vi "PIM Configuration.vi"(6 "Write? (f)":bool, 7 "Connection Refnum":T2, 8 "error in (no error)":errorcluster, 9 "Configuration (\"\")":string, 11 "Template Keys (empty)":T1) -> (0 "error out":errorcluster, 1 "Configuration":string, 3 "Template Keys":T1, 5 "Connection Refnum":T2)   [LabVIEW 2011]
uses:
  ITK/utils/keyedarr.llb/Keyed Array.ctl
  ITK/utils/strutil.llb/Case Matching.ctl
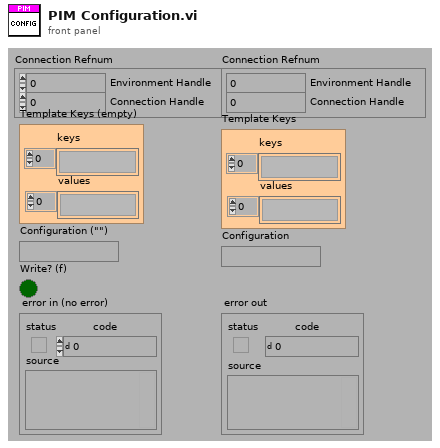
[diagram p1: front panel]
types:
  T1 = typedef "Keyed Array.ctl" = cluster{"keys":string[], "values":string[]}
  T2 = cluster{"Environment Handle":i32, "Connection Handle":i32}
  T3 = typedef "Case Matching.ctl" = enum16{"a != A", "a == A", "system"}
  T4 = typedef "PIM Test Parameters.ctl" = cluster{"Stimulus":T5, "Measure":T7, "Display":T13}
  T5 = typedef "PIM Stimulus Parameters.ctl" = cluster{"C1 Pwr dBm":dbl, "C2 Pwr dBm":dbl, "Power Units":enum16{"dBm", "Watts"}, "Meas Type":enum32{"Time", "Frequency"}, "C1 Freq MHz":dbl, "C2 Freq MHz":dbl, "Swept Freq Step":T6}
  T6 = typedef "PIM Sweep Step Size.ctl" = u16
  T7 = typedef "PIM Measurement Parameters.ctl" = cluster{"IM Order":T8, "Direction":T9, "Averaging":T10, "ALC ON?":bool, "Peak Hold?":bool, "Peak last N":u32, "Ref Level dBm":dbl, "Ref Units":enum16{"dBm", "dBc"}, "Num Samples":u32, "Sample units":T11, "Update Rate (s)":dbl, "DUT PORT":T12, "Percent (%)":u8}
  T8 = typedef "IMOrder.ctl" = u8
  T9 = typedef "MeasMode.ctl" = u16
  T10 = typedef "HW Averaging.ctl" = u16
  T11 = typedef "PIM Meas Units.ctl" = enum16{"Sample(s)", "Second(s)", "Sweep(s)"}
  T12 = typedef "DUTport.ctl" = enum16{"Port 1", "Port 2"}
  T13 = typedef "PIM Display Parameters.ctl" = cluster{"Power Scale":cluster{"yRange_min":i32, "yRange_max":i32}, "xRange_span":u32}
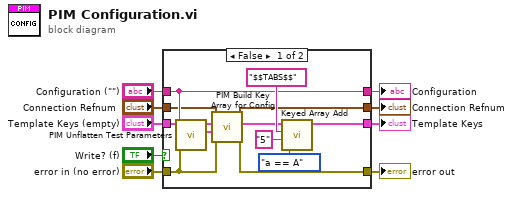
[diagram p0: block diagram]
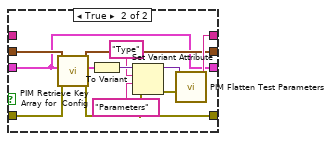
[diagram p2: hidden frame]
diagram:
  n1 = case shown="False" "Write? (f)" {
    tunnel: "error in (no error)" -> [w10 w27]
    tunnel: [w14 w22] -> w8
    tunnel: "Template Keys (empty)" -> [w12 w22]
    tunnel: "Configuration (\"\")" -> [w18 _]
    tunnel: [w13 w26] -> w5
    tunnel: [w18 w28] -> w4
    tunnel: "Connection Refnum" -> [w17 w25]
    tunnel: [w16 w24] -> w1
    frame False {
      n2 = call "PIM Unflatten Test Parameters.vi"("error in (no error)"=w10, "Parameter String"=w18) -> ("PIM Test Parameters"=w11:T4)  [unwired: 9 out]
      n3 = call "PIM Build Key Array for Config.vi"("error in (no error)"=w10, "PIM Test Parameters"=w11, "Key Array In"=w12, "Connection Refnum"=w17) -> ("error out"=w13:errorcluster, "Key Array Out"=w15:T1, "Connection Refnum"=w16:T2)  [unwired: 5 out]
      n4 = call "Keyed Array Add.vi"("case matching (sensitive)"=Case_Matching."a == A", "value"="5", "key"="$$TABS$$", "array in"=w15) -> ("array out"=w14:T1)  [unwired: 3 out]
    }
    frame True {
      n5 = call "PIM Retrieve Key Array for  Config.vi"("error in (no error)"=w27, "Key Array In"=w22, "Connection Refnum"=w25) -> ("error out"=w26:errorcluster, "PIM Test Parameters"=w23:T4, "Connection Refnum"=w24:T2)  [unwired: 1 in, 5 out]
      n6 = To Variant(anything=w23) -> (Variant=w33:variant)
      n7 = Set Variant Attribute(Variant=w33, name="Type", value="Parameters" ("name"), error in=w26) -> (Variant out=w29:variant, error out=w32:errorcluster)  [unwired: 1 out]
      n8 = call "PIM Flatten Test Parameters.vi"("error in (no error)"=w32, "Parameter Variant"=w29) -> ("Parameter String"=w28:string)  [unwired: 9 out]
    }
  }
  "error out" <- w5
  "Connection Refnum" <- w1
  "Template Keys" <- w8
  "Configuration" <- w4
